vi "_Check Option.vi"(6 "Error generation (Error if missing)":T1(ring), 8 "error in (no error)":errorcluster, 10 "Option":string, 11 "VISA resource name":refnum<visa-resource-name>) -> (0 "error out":errorcluster, 2 "Option installed":bool, 3 "VISA resource name out":refnum<visa-resource-name>)   [LabVIEW 2015, in "Rohde&Schwarz CMP LR WPAN Measurement.lvlib"]
doc: "This VI checks whether instrument is equipped with the entered option."
uses:
  <instrlib>/Rohde&Schwarz CMP LR WPAN Measurement/Rohde&Schwarz CMP LR WPAN Measurement.lvlib
  <instrlib>/Rohde&Schwarz CMP LR WPAN Measurement/Private/rsidr_core.llb/type_Attribute.ctl
  <instrlib>/Rohde&Schwarz CMP LR WPAN Measurement/Private/rsidr_core.llb/type_Attribute_Data_Type.ctl
  <instrlib>/Rohde&Schwarz CMP LR WPAN Measurement/Private/rsidr_core.llb/type_ReadWriteAccess.ctl
  <instrlib>/Rohde&Schwarz CMP LR WPAN Measurement/Private/rsidr_core.llb/rsidr_core.lvlib
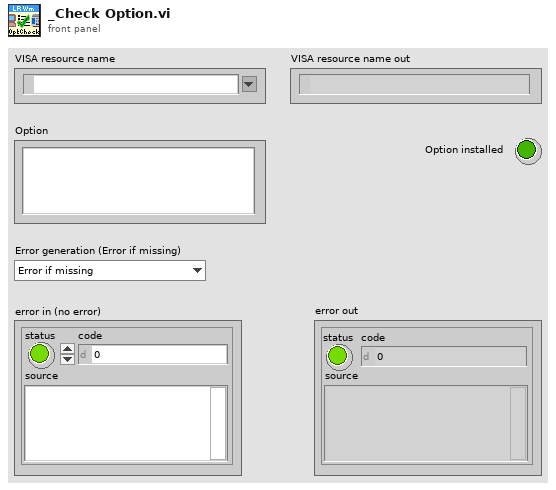
[diagram p1: front panel]
types:
  T1 = enum16{"Error if missing", "Error if present", "No error"}
  T2 = typedef "Rohde&Schwarz CMP LR WPAN Measurement.lvlib/rsidr_core.lvlib/type_Attribute.ctl" = cluster{"Identifier":string, "Descriptive Name":string, "Data Type":T3, "Command":string, "Access":T4, "Range Table":string, "Read Callback":string, "Write Callback":string, "Supported Models":string, "Instrument Options":string, "Index":i32, "OPC Wait":bool, "No Status Check":bool, "Cache Only":bool}
  T3 = typedef "Rohde&Schwarz CMP LR WPAN Measurement.lvlib/rsidr_core.lvlib/type_Attribute_Data_Type.ctl" = enum16{"Integer 32", "Double", "String", "Boolean", "None", "Integer 64", "RawString"}
  T4 = typedef "Rohde&Schwarz CMP LR WPAN Measurement.lvlib/rsidr_core.lvlib/type_ReadWriteAccess.ctl" = enum16{"Read Only", "Write Only", "Read/Write"}
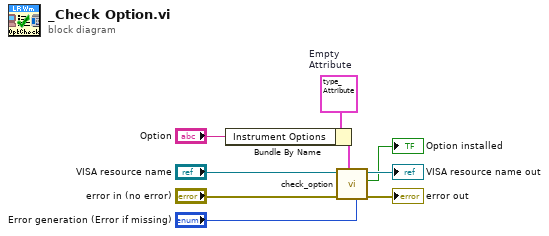
[diagram p0: block diagram]
diagram:
  w3 = T2 {"Identifier"="", "Descriptive Name"="", "Data Type"=enum."Integer 32", "Command"="", "Access"=enum."Read/Write", "Range Table"="", "Read Callback"="", "Write Callback"="", "Supported Models"="", "Instrument Options"="", "Index"=0, "OPC Wait"=FALSE, "No Status Check"=FALSE, "Cache Only"=FALSE}  # Empty Attribute
  n1 = Bundle By Name(cluster=w3, "Instrument Options"="Option") -> (w4:T2)
  n2 = call <instrlib>:"check_option.vi"("Error generation (Error if missing)"="Error generation (Error if missing)", "Attribute"=w4, "error in"="error in (no error)", "VISA resource name"="VISA resource name") -> ("error out"=→"error out":errorcluster, "Option installed"=→"Option installed":bool, "VISA resource name out"=→"VISA resource name out":refnum<visa-resource-name>)  [unwired: 5 in]
